vi "deregister.vi"(0 "HGF_Monitor in":refnum<class "HGF_Monitor.lvclass">, 1 "Variable":string, 2 "HGF_NetworkVisitor":refnum<class "HGF_NetworkVisitor.lvclass">, 3 "HGF_TriggeredEvent":refnum<class "HGF_TriggeredEvent.lvclass">, 4 "Rem SV/Visitor from List":bool, 5 "error in (no error)":errorcluster) -> (14 "HGF_Monitor out":refnum<class "HGF_Monitor.lvclass">, 19 "error out":errorcluster)   [LabVIEW 2012, in "HGF_SV.lvlib" / "HGF_Monitor.lvclass"]
uses:
  HGF_Monitor.lvclass
  HGF_BaseClasses/HGF_TriggeredEvent/HGF_TriggeredEvent.lvclass
  HGF_BaseClasses/HGF_NetworkVisitor/HGF_NetworkVisitor.lvclass
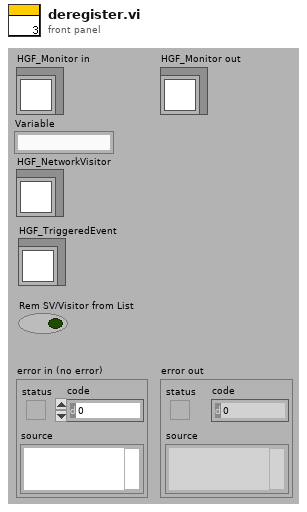
[diagram p1: front panel]
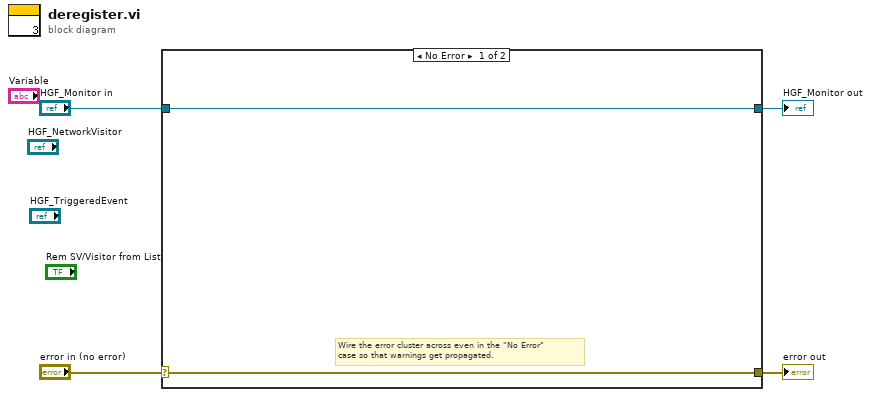
[diagram p0: block diagram]
diagram:
  n1 = case shown="No Error" "error in (no error)" {
    selector: "error in (no error)" -> [w5 w8]
    tunnel: [w5 w8] -> w3
    tunnel: [w6 w7] -> w1
    tunnel: "HGF_Monitor in" -> [w6 w7]
    frame No Error {
      # "Wire the error cluster across even in the \"No Error\"\ncase so that warnings get propagated."
    }
    frame Error {
    }
  }
  "error out" <- w3
  "HGF_Monitor out" <- w1
